vi "Queue Create.vi"(9 "Queue Actor":refnum<class "Queue Actor.lvclass">, 10 "Alias":string, 11 "Hello World Queue in":refnum<class "Hello World Queue.lvclass">) -> (3 "Hello World Queue out":refnum<class "Hello World Queue.lvclass">)   [LabVIEW 2021, in "Hello World Queue.lvlib" / "Hello World Queue.lvclass"]
uses:
  Hello World Queue.lvclass
  jettl/jettl/Queue Actor/Queue Actor.lvclass
  Hello World Queue.lvclass/Hello World Queue.ctl
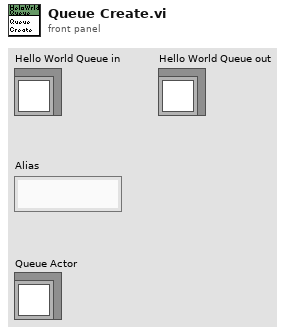
[diagram p1: front panel]
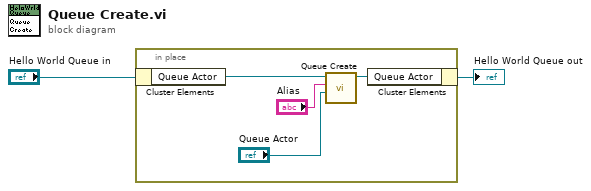
[diagram p0: block diagram]
diagram:
  n1 = in-place {
    n2 = in-place-cluster #1("Hello World Queue in") -> ("Queue Actor"=w4:refnum<class "Queue Actor.lvclass">)
    n3 = call-dynamic "Queue Create.vi"("Queue Actor"="Queue Actor", "Alias"="Alias", "Queue Create in"=w4) -> ("Queue Create out"=w3:refnum<class "Queue Actor.lvclass">)  [unwired: 8 in]
    n4 = in-place-cluster #1("Queue Actor"=w3) -> (→"Hello World Queue out":refnum<class "Hello World Queue.lvclass">)
  }
